vi "Get Time.vi"() -> (3 "Time in Seconds":dbl)   [LabVIEW 2019]
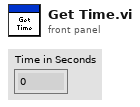
[diagram p1: front panel]
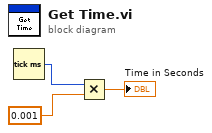
[diagram p0: block diagram]
diagram:
  n1 = Tick Count (ms)() -> (millisecond timer value=w2:u32)
  n2 = Multiply(x=w2, y=0.001) -> (x*y=→"Time in Seconds":dbl)
